vi "Get Checksum.vi"(10 "Input":string) -> (2 "Checksum":string)   [LabVIEW 2018, in "TE Cooler.lvlib" / "TE Cooler.lvclass"]
doc: "Calculate the checksum for the command to be sent. From the manual:\n\nThe 8]bit (modulo 256) hexadecimal checksum of characters sent to/from the controlling computer. This is represented as 2 ASCII characters. The checksum calculation excludes the characters (stx), SS, and (etx). The TC]36]25 RS232 sums (in an 8]bit register) the hexadecimal values of the ASCII characters sent to/from the controlling computer. Any overflow is truncated, leaving the 8]bit (modulo 256) checksum. When the controller is receiving data, this controller calculates the checksum and compares it to the checksum sent by the controlling computer. The TC]36]25 RS232 will respond as shown below depending on whether or not the checksums match. When the controlling computer is receiving data the checksum sent by the controller can be used to make sure the data has not been received with an error. Remember, when finding the ASCII value for a hexadecimal number (a, b, c, d, e, and f) be sure to reference lower case letters."
uses:
  TE Cooler.lvclass
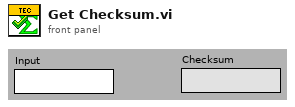
[diagram p1: front panel]
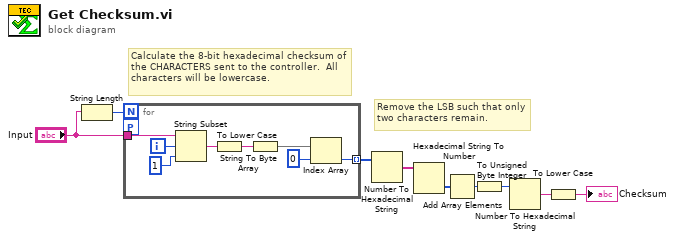
[diagram p0: block diagram]
diagram:
  # "Calculate the 8-bit hexadecimal checksum of the CHARACTERS sent to the controller.  All characters will be lowercase."
  # "Remove the LSB such that only two characters remain."
  n1 = String Length(string="Input") -> (length=w1:i32)
  n2 = for {
    N: w1 -> [_]
    tunnel: "Input" -> [w17]
    tunnel: [w14] -> w2 mode=indexing
    workers-P: _ -> [_]
    i -> [w16]
    n3 = String Subset(string=w17, offset (0)=w16, length (rest)=1 ("length (rest)")) -> (substring=w10:string)
    n4 = To Lower Case(string=w10) -> (all lower case string=w11:string)
    n5 = String To Byte Array(string=w11) -> (unsigned byte array=w13:u8[])
    n6 = Index Array(array=w13, index=0) -> (element=w14:u8)
  }
  n7 = Number To Hexadecimal String(2:w2) -> (0:w3:string[])  [unwired: 1 out]
  n8 = Hexadecimal String To Number(string=w3) -> (number=w4:u32[])  [unwired: 3 out]
  n9 = Add Array Elements(numeric array=w4) -> (sum=w5:u32)
  n10 = To Unsigned Byte Integer(number=w5) -> (unsigned 8bit integer=w6:u8)
  n11 = Number To Hexadecimal String(2:w6) -> (0:w7:string)  [unwired: 1 out]
  n12 = To Lower Case(string=w7) -> (all lower case string=→"Checksum":string)
